vi "RMX41xInit.vi"(0 "VISA resource name":refnum<visa-resource-name>, 3 "error in (no error)":errorcluster) -> (5 "resulting string":string, 6 "DeviceErrorCode":i32, 7 "VISA resource name out":refnum<visa-resource-name>, 8 "Status":i32, 9 "Error":bool, 10 "error out 2":errorcluster)   [LabVIEW 2023]
panel:
  out "RMXInformation":string
  out "Instrument Firmware Revision":string
  out "Instrument Driver Revision":string
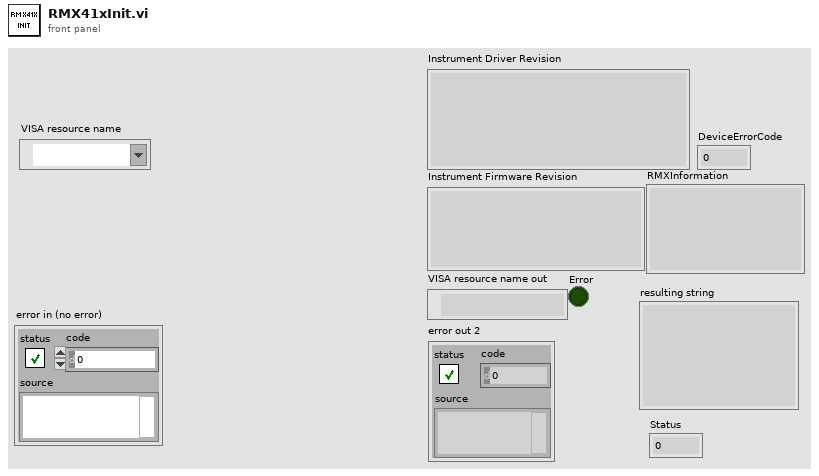
[diagram p1: front panel]
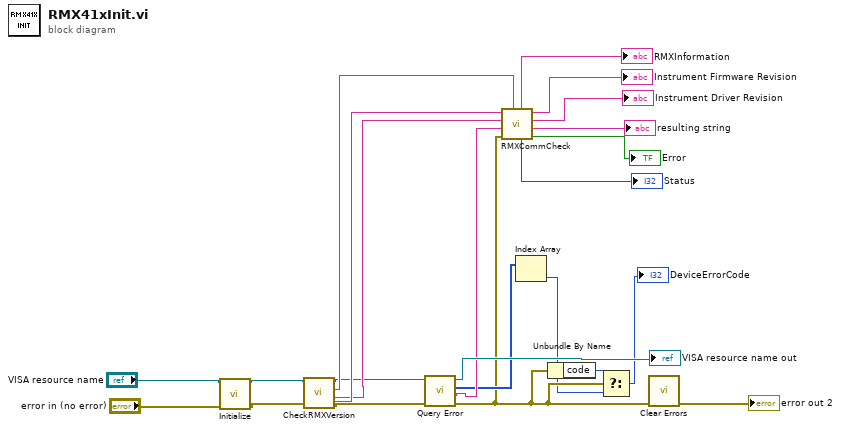
[diagram p0: block diagram]
diagram:
  n1 = call "Initialize.vi"("error in (no error)"="error in (no error)", "VISA resource name"="VISA resource name") -> ("error out"=w11:errorcluster, "VISA resource name out"=w10:refnum<visa-resource-name>)  [unwired: 8 in]
  n2 = call "CheckRMXVersion.vi"("error in (no error)"=w11, "VISA resource name"=w10) -> ("error out"=w8:errorcluster, "Instrument Driver Revision"=w21:string, "Instrument Firmware Revision"=w22:string, "VISA resource name out"=w9:refnum<visa-resource-name>, "RMXInformation"=w23:string)  [unwired: 5 in]
  n3 = call "Query Error.vi"("error in (no error)"=w8, "VISA resource name"=w9) -> ("error out"=w4:errorcluster, "Error Message"=w6:string, "Error Code"=w5:i32[], "VISA resource name out"=→"VISA resource name out":refnum<visa-resource-name>)  [unwired: 6 in]
  n4 = call "RMXCommCheck.vi"("Instrument Firmware Revision in"=w22, "error in (no error)"=w4, "Error Message"=w6, "Instrument Driver Revision in"=w21, "RMXInformation in"=w23) -> ("Error"=→"Error":bool, "resulting string"=→"resulting string":string, "Instrument Driver Revision out"=→"Instrument Driver Revision":string, "Instrument Firmware Revision out"=→"Instrument Firmware Revision":string, "f"=→"Status":i32, "RMXInformation out"=→"RMXInformation":string)  [unwired: 1 in]
  n5 = Index Array(array=w5) -> (element=w2:i32)  [unwired: 1 in]
  n6 = Unbundle By Name(w4) -> ("code"=w3:i32)
  n7 = Select(t=w3, s=w4, f=w2) -> (s? t:f=→"DeviceErrorCode":i32)
  n8 = call <vilib>:"Clear Errors.vi"("error in (no error)"=w4) -> ("error out"=→"error out 2":errorcluster)  [unwired: 5 in, 1 out]
